vi "test Add Get and Remove Timestamp Channel.vi"(8 "error in":errorcluster, 11 "TestCase in":refnum<class "Scripting.lvclass">) -> (0 "error out":errorcluster, 3 "TestCase out":refnum<class "Scripting.lvclass">)   [LabVIEW 2020, in "Scripting.lvclass"]
uses:
  Scripting.lvclass
  <vilib>/NI VeriStand/Custom Device API/Custom Device Item Ref.ctl
  Scripting.lvclass/Scripting.ctl
  <vilib>/addons/_JKI Toolkits/VI Tester/TestCase.llb/TestCase.lvclass
  Scripting/Ballard/Ballard ARINC 429 Scripting.lvlib
  <vilib>/NI VeriStand/Custom Device API/Custom Device API.lvlib
  C:/Program Files (x86)/National Instruments/LabVIEW 2020/vi.lib/addons/_JKI Toolkits/VI Tester/TestCase.llb/TestCase.lvclass
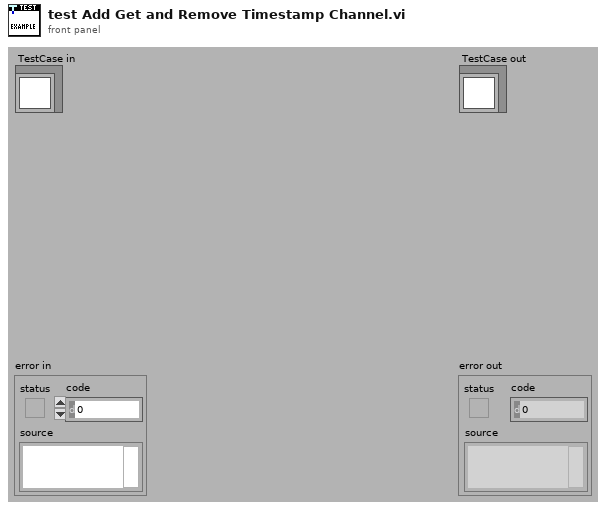
[diagram p1: front panel]
types:
  T1 = typedef "Custom Device API.lvlib/Custom Device Item Ref.ctl" = u64
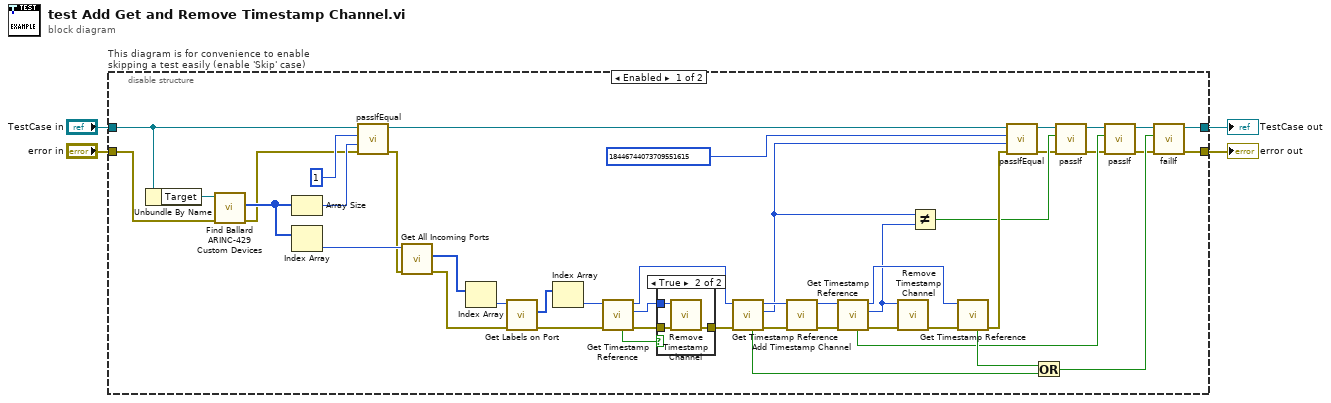
[diagram p0: block diagram]
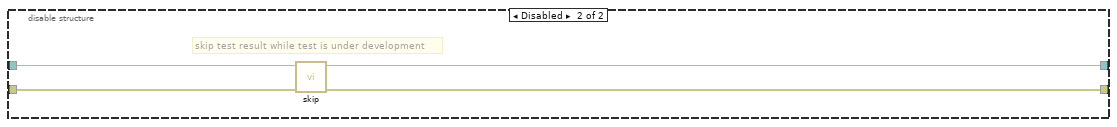
[diagram p3: hidden frame]
diagram:
  n1 = disable-structure "This diagram is for convenience to enable skipping a test easily (enable 'Skip' case)" shown="Enabled" {
    disable-tunnel: "TestCase in" -> [w47 w57]
    disable-tunnel: [w12 w55] -> w1
    disable-tunnel: [w13 w56] -> w3
    disable-tunnel: "error in" -> [w46 w54]
    frame Enabled {
      n2 = Unbundle By Name(w47) -> ("Target"=w49:refnum<k24>)
      n3 = call "Find Ballard ARINC-429 Custom Devices.vi"("error in"=w46, "target in"=w49) -> ("error out"=w37:errorcluster, "Ballard ARINC 429 custom devices"=w39:u64[])  [unwired: 7 in, 1 out]
      n4 = Array Size(array=w39) -> (size(s)=w44:i32)
      n5 = Index Array(array=w39) -> (element=w48:u64)  [unwired: 1 in]
      n6 = call-dynamic "passIfEqual.vi"("error in (no error)"=w37, "y"=w44, "x"=1 ("size(s)"), "TestCase in"=w47) -> ("error out"=w36:errorcluster, "TestCase out"=w38:refnum<class "Scripting.lvclass">)  [unwired: 6 in]
      n7 = call "Get All Incoming Ports.vi"("error in"=w36, "Ballard ARINC 429 ref"=w48) -> ("error out"=w41:errorcluster, "Port refs"=w43:T1[])  [unwired: 7 in, 1 out]
      n8 = Index Array(array=w43) -> (element=w42:T1)  [unwired: 1 in]
      n9 = call "Get Labels on Port.vi"("error in"=w41, "port ref"=w42) -> ("error out"=w19:errorcluster, "label references"=w40:T1[])  [unwired: 6 in, 2 out]
      n10 = Index Array(array=w40) -> (element=w20:T1)  [unwired: 1 in]
      n11 = call "Get Timestamp Reference.vi"("error in"=w19, "label ref in"=w20) -> ("error out"=w18:errorcluster, "timestamp channel reference"=w21:T1, "label ref out"=w17:T1, "timestamp channel found?"=w5:bool)  [unwired: 6 in]
      n12 = case shown="True" w5 {
        tunnel: w21 -> [_ w53]
        tunnel: w18 -> [w50 w52]
        tunnel: [w50 w51] -> w6
        frame False {
        }
        frame True {
          n13 = call "Remove Timestamp Channel.vi"("error in"=w52, "timestamp channel ref"=w53) -> ("error out"=w51:errorcluster)  [unwired: 9 in]
        }
      }
      n14 = call "Get Timestamp Reference.vi"("error in"=w6, "label ref in"=w17) -> ("error out"=w34:errorcluster, "timestamp channel reference"=w25:T1, "label ref out"=w35:T1, "timestamp channel found?"=w15:bool)  [unwired: 6 in]
      n15 = call "Add Timestamp Channel.vi"("error in"=w34, "label ref"=w35) -> ("error out"=w32:errorcluster, "label ref out"=w33:T1)  [unwired: 8 in]
      n16 = call "Get Timestamp Reference.vi"("error in"=w32, "label ref in"=w33) -> ("error out"=w30:errorcluster, "timestamp channel reference"=w26:T1, "label ref out"=w31:T1, "timestamp channel found?"=w11:bool)  [unwired: 6 in]
      n17 = call "Remove Timestamp Channel.vi"("error in"=w30, "timestamp channel ref"=w26) -> ("error out"=w29:errorcluster)  [unwired: 9 in]
      n18 = Not Equal?(x=w25, y=w26) -> (x != y?=w24:bool)
      n19 = call "Get Timestamp Reference.vi"("error in"=w29, "label ref in"=w31) -> ("error out"=w27:errorcluster, "timestamp channel found?"=w16:bool)  [unwired: 6 in, 2 out]
      n20 = call-dynamic "passIfEqual.vi"("error in (no error)"=w27, "y"=w25, "x"=T1 18446744073709551615 ("timestamp channel reference"), "TestCase in"=w38) -> ("error out"=w22:errorcluster, "TestCase out"=w23:refnum<class "Scripting.lvclass">)  [unwired: 6 in]
      n21 = Or(x=w16, y=w15) -> (x .or. y?=w14:bool)
      n22 = call-dynamic "passIf.vi"("error in (no error)"=w22, "pass"=w24, "TestCase in"=w23) -> ("error out"=w9:errorcluster, "TestCase out"=w10:refnum<class "Scripting.lvclass">)  [unwired: 7 in]
      n23 = call-dynamic "passIf.vi"("error in (no error)"=w9, "pass"=w11, "TestCase in"=w10) -> ("error out"=w7:errorcluster, "TestCase out"=w8:refnum<class "Scripting.lvclass">)  [unwired: 7 in]
      n24 = call-dynamic "failIf.vi"("error in (no error)"=w7, "fail"=w14, "TestCase in"=w8) -> ("error out"=w13:errorcluster, "TestCase out"=w12:refnum<class "Scripting.lvclass">)  [unwired: 7 in]
    }
    frame Disabled {
      # "skip test result while test is under development"
      n25 = call <vilib>:"skip.vi"("error in (no error)"=w54, "TestCase in"=w57) -> ("error out"=w56:errorcluster, "TestCase out"=w55:refnum<class "Scripting.lvclass">)  [unwired: 8 in]
    }
  }
  "error out" <- w3
  "TestCase out" <- w1
